vi "Run.vi"(9 "Team In":refnum<class "Team.lvclass">, 11 "MySquare in":refnum<class "MySquare.lvclass">) -> (1 "Team":refnum<class "Team.lvclass">, 2 "Run Result":T1={"Action"=enum."Move", "Direction"=enum."NW", "Replication"=refnum}, 3 "Square out":refnum<class "Square.lvclass">)   [LabVIEW 2020, in "The_Hill_Youth.lvlib" / "MySquare.lvclass"]
doc: "This VI is called on every active square each turn of the game for the square to decide what action to take."
uses:
  MySquare.lvclass
  C:/dev/lv20CE/sol-squarebattle/ProjectTemplates/Source/SummerOfLabVIEW/SquareBattle/template/SquareBattle/Square/Square.lvclass
  SquareBattle/Square/Square.lvclass
  SquareBattle/Run Result.ctl
  SquareBattle/Action.ctl
  SquareBattle/Direction.ctl
  SquareBattle/Team/Team.lvclass
  MyTeam/MyTeam.lvclass
  C:/dev/lv20CE/sol-squarebattle/ProjectTemplates/Source/SummerOfLabVIEW/SquareBattle/template/SquareBattle/Team/Team.lvclass
  SquareBattle/Square/Square.lvclass/Square.ctl
  MyTeam/map_point.ctl
  MySquare.lvclass/MySquare.ctl
  SquareBattle/Team/Team.lvclass/Team.ctl
  SquareBattle/SquareBattle.lvlib
  The_Hill_Youth.lvlib
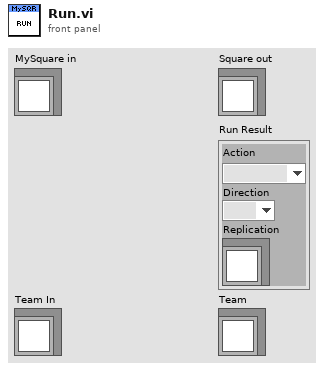
[diagram p1: front panel]
types:
  T1 = typedef "SquareBattle.lvlib/Run Result.ctl" = cluster{"Action":T2, "Direction":T3, "Replication":refnum<class "Square.lvclass">}
  T2 = typedef "SquareBattle.lvlib/Action.ctl" = enum16{"Wait", "Move", "Attack", "Replicate"}
  T3 = typedef "SquareBattle.lvlib/Direction.ctl" = enum16{"NW", "N", "NE", "E", "SE", "S", "SW", "W"}
  T4 = typedef "The_Hill_Youth.lvlib/map_point.ctl" = cluster{"status":enum16{"unknown", "frind", "enemy", "empty"}, "plans":enum16{"stay", "duplicate", "attack", "move to", "no plans"}, "age":dbl}
  T5 = typedef "SquareBattle.lvlib/Position.ctl" = cluster{"Row":i32, "Col":i32}
  T6 = enum16{"stay", "duplicate", "attack", "move to", "no plans"}
  T7 = typedef "SquareBattle.lvlib/Team Stats.ctl" = cluster{"Active":i32, "Generated":i32, "Kills":i32, "Eliminated":i32, "Collided":i32}
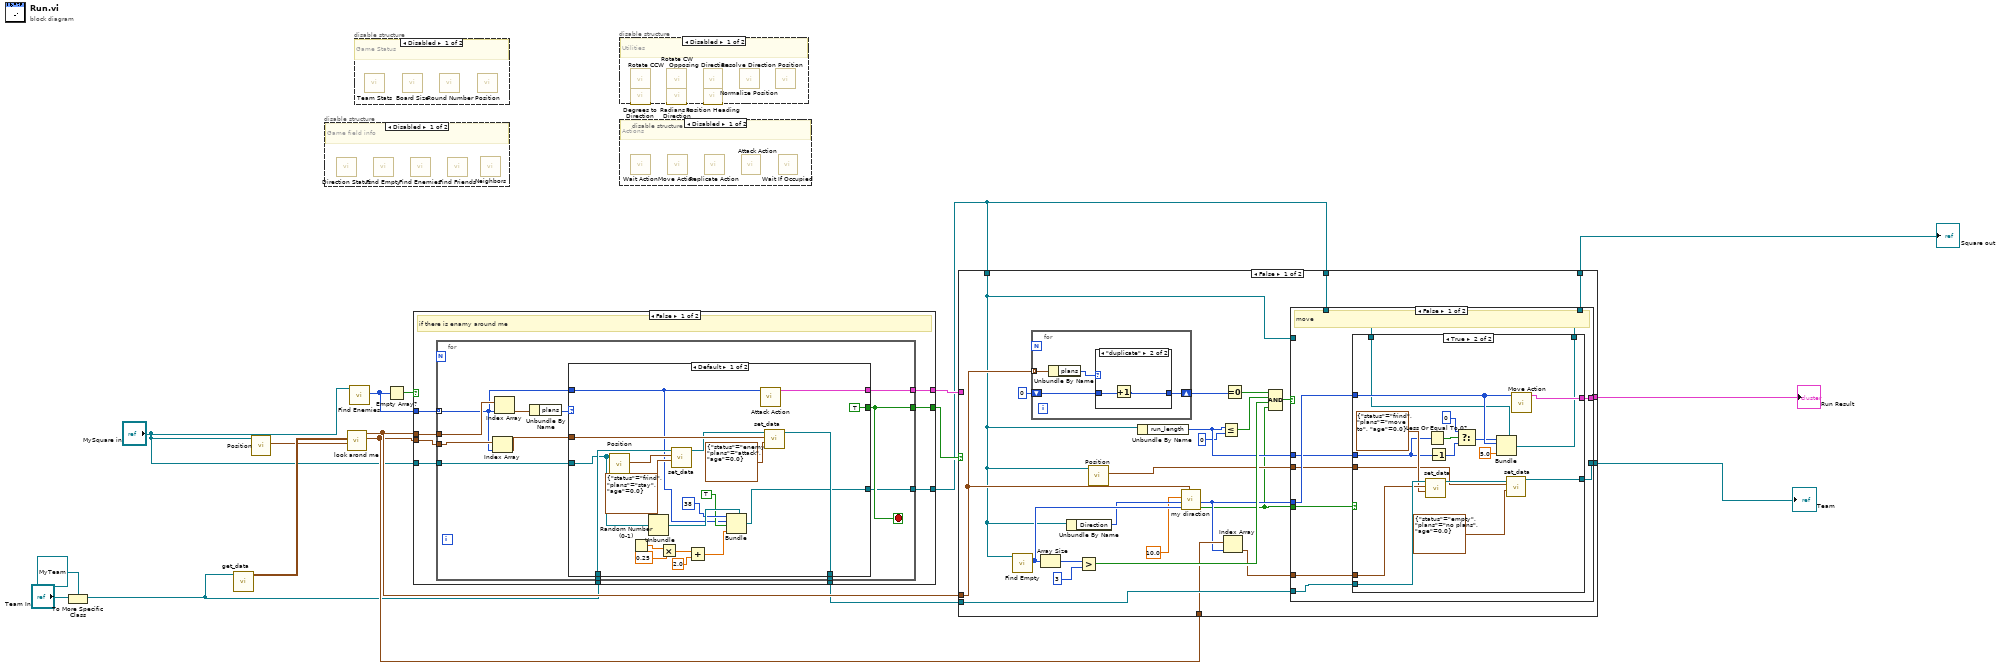
[diagram p0: block diagram]
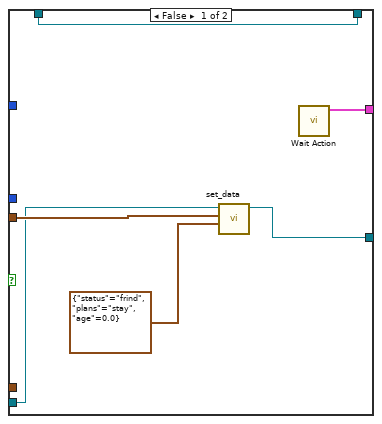
[diagram p2: hidden frame]
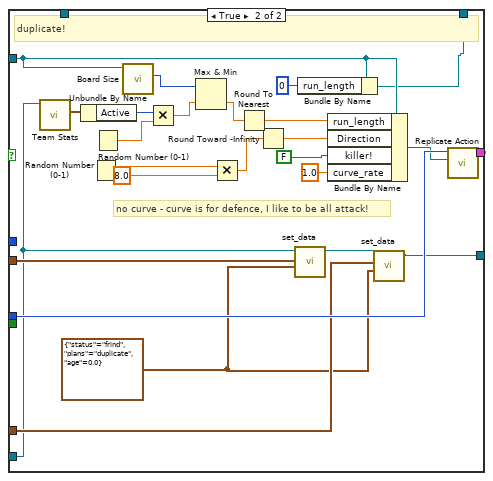
[diagram p3: hidden frame]
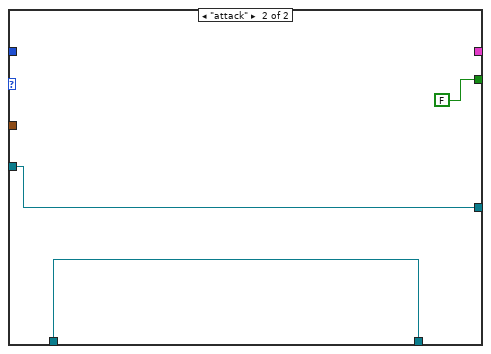
[diagram p6: hidden frame]
diagram:
  n1 = To More Specific Class(target class=refnum<class "MyTeam.lvclass"> refnum ("SquareTeam.lvlib:MyTeam.lvclass"), reference="Team In") -> (specific class reference=w7:refnum<class "MyTeam.lvclass">)  [unwired: 1 in, 1 out]
  n2 = call "get_data.vi"("SquareTeam.lvlib:MyTeam.lvclass"=w7) -> ("map"=w15:T4[][])  [unwired: 9 in, 1 out]
  n3 = call "Position.vi"("Square in"="MySquare in") -> ("Position"=w4:T5)  [unwired: 10 in]
  n4 = disable-structure shown="Disabled" {
    frame Disabled {
      # "Game field info"
      n5 = call "Direction Status.vi"() -> ()  [unwired: 10 in, 2 out]
      n6 = call "Find Empty.vi"() -> ()  [unwired: 11 in, 1 out]
      n7 = call "Find Enemies.vi"() -> ()  [unwired: 11 in, 1 out]
      n8 = call "Find Friends.vi"() -> ()  [unwired: 11 in, 1 out]
      n9 = call "Neighbors.vi"() -> ()  [unwired: 11 in, 1 out]
    }
    frame Enabled {
    }
  }
  n10 = call "look arond me.vi"("Position"=w4, "map"=w15) -> ("index_out"=w8:cluster{"Numeric":i32, "Numeric":i32}[], "map data of it"=w11:T4[])  [unwired: 8 in]
  n11 = call "Find Enemies.vi"("Square"="MySquare in") -> ("Enemy Directions"=w13:T3[])  [unwired: 10 in]
  n12 = disable-structure shown="Disabled" {
    frame Disabled {
      # "Game Status"
      n13 = call "Team Stats.vi"() -> ()  [unwired: 11 in, 1 out]
      n14 = call "Board Size.vi"() -> ()  [unwired: 11 in, 1 out]
      n15 = call "Round Number.vi"() -> ()  [unwired: 11 in, 1 out]
      n16 = call "Position.vi"() -> ()  [unwired: 11 in, 1 out]
    }
    frame Enabled {
    }
  }
  n17 = Empty Array?(array=w13) -> (empty?=w14:bool)
  n18 = case shown="False" w14 {
    tunnel: w13 -> [w26 _]
    tunnel: w11 -> [w25 _]
    tunnel: w8 -> [w24 _]
    tunnel: w7 -> [w23 w62]
    tunnel: [w22 _] -> w12
    tunnel: [w21 _] -> w10
    tunnel: [w20 w62] -> w9
    tunnel: "MySquare in" -> [w19 w61]
    tunnel: [w18 w61] -> w5
    frame False {
      # "if there is enamy around me"
      n19 = for {
        tunnel: w26 -> [w34] mode=indexing
        tunnel: w25 -> [w38]
        tunnel: w24 -> [w35]
        tunnel: w23 -> [w32]
        tunnel: [w31] -> w22
        tunnel: [w30] -> w21
        tunnel: [w29] -> w20
        tunnel: w19 -> [w27]
        tunnel: [w28] -> w18
        stop <- w30 stop-if-true
        n20 = Index Array(array=w35, index=w34) -> (element=w33:cluster{"Numeric":i32, "Numeric":i32})
        n21 = Index Array(array=w38, index=w34) -> (element=w37:T4)
        n22 = Unbundle By Name(w37) -> ("plans"=w36:T6)
        n23 = case shown="Default" w36 {
          tunnel: [TRUE FALSE] -> w30
          tunnel: w34 -> [w44 _]
          tunnel: [w56 _] -> w31
          tunnel: w33 -> [w55 _]
          tunnel: w32 -> [w53 w59]
          tunnel: [w49 w59] -> w29
          tunnel: w27 -> [w48 w58]
          tunnel: [w47 w58] -> w28
          frame Default {
            n24 = call "Position.vi"("Square in"=w48) -> ("Position"=w51:T5)  [unwired: 10 in]
            n25 = Random Number (0-1)() -> (number: 0 to 1=w43:dbl)
            n26 = Unbundle(w48) -> ()  [unwired: 4 out]
            n27 = Multiply(x=w43, y=0.25) -> (x*y=w42:dbl)
            n28 = call "set_data.vi"("new data"=T4 {"status"=enum."frind", "plans"=enum."stay", "age"=0.0}, "point to set index"=w51, "SquareTeam.lvlib:MyTeam.lvclass 2"=w53) -> ("SquareTeam.lvlib:MyTeam.lvclass"=w52:refnum<class "MyTeam.lvclass">)  [unwired: 8 in]
            n29 = Add(x=w42, y=2.0) -> (x+y=w40:dbl)
            n30 = Bundle(cluster=w48, 38 ("x"), w44, TRUE ("killer!"), w40) -> (w47:refnum<class "MySquare.lvclass">)
            n31 = call "Attack Action.vi"("Direction"=w44) -> ("Run Result"=w56:T1)  [unwired: 10 in]
            n32 = call "set_data.vi"("new data"=T4 {"status"=enum."enemy", "plans"=enum."attack", "age"=0.0}, "point to set index"=w55, "SquareTeam.lvlib:MyTeam.lvclass 2"=w52) -> ("SquareTeam.lvlib:MyTeam.lvclass"=w49:refnum<class "MyTeam.lvclass">)  [unwired: 8 in]
          }
          frame "attack" {
          }
        }
      }
    }
    frame True {
    }
  }
  n33 = disable-structure shown="Disabled" {
    frame Disabled {
      # "Utilities"
      n34 = call "Rotate CCW.vi"() -> ()  [unwired: 11 in, 1 out]
      n35 = call "Degrees to Direction.vi"() -> ()  [unwired: 11 in, 1 out]
      n36 = call "Rotate CW.vi"() -> ()  [unwired: 11 in, 1 out]
      n37 = call "Radians to Direction.vi"() -> ()  [unwired: 11 in, 1 out]
      n38 = call "Opposing Direction.vi"() -> ()  [unwired: 11 in, 1 out]
      n39 = call "Position Heading.vi"() -> ()  [unwired: 10 in, 2 out]
      n40 = call "Normalize Position.vi"() -> ()  [unwired: 10 in, 2 out]
      n41 = call "Resolve Direction Position.vi"() -> ()  [unwired: 9 in, 3 out]
    }
    frame Enabled {
    }
  }
  n42 = disable-structure shown="Disabled" {
    frame Disabled {
      # "Actions"
      n43 = call "Wait Action.vi"() -> ()  [unwired: 11 in, 1 out]
      n44 = call "Move Action.vi"() -> ()  [unwired: 11 in, 1 out]
      n45 = call "Replicate Action.vi"() -> ()  [unwired: 11 in, 1 out]
      n46 = call "Attack Action.vi"() -> ()  [unwired: 11 in, 1 out]
      n47 = call "Wait If Occupied.vi"() -> ()  [unwired: 11 in, 1 out]
    }
    frame Enabled {
    }
  }
  n48 = case shown="False" w10 {
    tunnel: w12 -> [_ w155]
    tunnel: [w77 w155] -> w3
    tunnel: w11 -> [w84 _]
    tunnel: w5 -> [w65 _]
    tunnel: w9 -> [w76 w154]
    tunnel: w5 -> [w75 w153]
    tunnel: w8 -> [w73 _]
    tunnel: [w71 w154] -> w6
    tunnel: [w70 w153] -> w1
    frame False {
      n49 = call "Find Empty.vi"("Square"=w65) -> ("Empty Directions"=w85:T3[])  [unwired: 10 in]
      n50 = for {
        tunnel: w84 -> [w149] mode=indexing
        shift-right: [w147] -> w82
        shift-left: u8 0 -> [w146]
        n51 = Unbundle By Name(w149) -> ("plans"=w148:T6)
        n52 = case shown="\"duplicate\"" w148 {
          tunnel: [w150 w152] -> w147
          tunnel: w146 -> [w150 w151]
          frame "stay", Default {
          }
          frame "duplicate" {
            n53 = Increment(x=w151) -> (x+1=w152:u8)
          }
        }
      }
      n54 = Array Size(array=w85) -> (size(s)=w87:i32)
      n55 = Unbundle By Name(w65) -> ("Direction"=w66:T3)
      n56 = Greater?(x=w87, y=3) -> (0:w79:bool)
      n57 = call "Position.vi"("Square in"=w65) -> ("Position"=w74:T5)  [unwired: 10 in]
      n58 = Unbundle By Name(w65) -> ("run_length"=w69:i32)
      n59 = call "my diraction.vi"(7:w84, "Empty Directions"=w85, "my diraction"=w66, "curve_rate"=10.0) -> ("you may act"=w64:bool, "Direction for act"=w67:i16)  [unwired: 5 in, 1 out]
      n60 = Less Or Equal?(x=w69, y=0) -> (x <= y?=w80:bool)
      n61 = Index Array(array=w73, index=w67) -> (element=w72:cluster{"Numeric":i32, "Numeric":i32})
      n62 = Equal To 0?(x=w82) -> (x = 0?=w81:bool)
      n63 = Compound Arithmetic op=AND(w81, w80, w79, w64) -> (w78:bool)
      n64 = case shown="False" w78 {
        tunnel: w67 -> [w96 w145]
        tunnel: [w95 w144] -> w77
        tunnel: w76 -> [w94 w130]
        tunnel: w75 -> [w89 _]
        tunnel: w74 -> [w91 w141]
        tunnel: w72 -> [w93 w139]
        tunnel: [w92 w137] -> w71
        tunnel: w64 -> [w97 _]
        tunnel: w69 -> [w90 _]
        tunnel: [w88 w124] -> w70
        tunnel: w65 -> [_ w125]
        frame False {
          # "move"
          n65 = case shown="True" w97 {
            tunnel: w96 -> [_ w111]
            tunnel: [w99 w120] -> w95
            tunnel: w94 -> [w102 w119]
            tunnel: w93 -> [_ w118]
            tunnel: [w100 w115] -> w92
            tunnel: w91 -> [w103 w114]
            tunnel: w90 -> [_ w110]
            tunnel: w89 -> [w98 w105]
            tunnel: [w98 w112] -> w88
            frame False {
              n66 = call "set_data.vi"("new data"=T4 {"status"=enum."frind", "plans"=enum."stay", "age"=0.0}, "point to set index"=w103, "SquareTeam.lvlib:MyTeam.lvclass 2"=w102) -> ("SquareTeam.lvlib:MyTeam.lvclass"=w100:refnum<class "MyTeam.lvclass">)  [unwired: 8 in]
              n67 = call "Wait Action.vi"() -> ("Run Result"=w99:T1)  [unwired: 11 in]
            }
            frame True {
              # "move!"
              n68 = call "set_data.vi"("new data"=T4 {"status"=enum."frind", "plans"=enum."move to", "age"=0.0}, "point to set index"=w118, "SquareTeam.lvlib:MyTeam.lvclass 2"=w119) -> ("SquareTeam.lvlib:MyTeam.lvclass"=w116:refnum<class "MyTeam.lvclass">)  [unwired: 8 in]
              n69 = Less Or Equal To 0?(x=w110) -> (x <= 0?=w108:bool)
              n70 = Decrement(x=w110) -> (x-1=w109:i32)
              n71 = Select(t=0, s=w108, f=w109) -> (s? t:f=w106:i32)
              n72 = Bundle(cluster=w105, w106, w111, 5.0 ("curve_rate")) -> (w112:refnum<class "MySquare.lvclass">)  [unwired: 1 in]
              n73 = call "set_data.vi"("new data"=T4 {"status"=enum."empty", "plans"=enum."no plans", "age"=0.0}, "point to set index"=w114, "SquareTeam.lvlib:MyTeam.lvclass 2"=w116) -> ("SquareTeam.lvlib:MyTeam.lvclass"=w115:refnum<class "MyTeam.lvclass">)  [unwired: 8 in]
              n74 = call "Move Action.vi"("Direction"=w111) -> ("Run Result"=w120:T1)  [unwired: 10 in]
            }
          }
        }
        frame True {
          w138 = T4 {"status"=enum."frind", "plans"=enum."duplicate", "age"=0.0} ("new data")
          # "no curve - curve is for defence, I like to be all attack!"
          # "duplicate!"
          n75 = call "Team Stats.vi"("Team"=w130) -> ("Team Stats"=w143:T7)  [unwired: 10 in]
          n76 = Unbundle By Name(w143) -> ("Active"=w123:i32)
          n77 = Random Number (0-1)() -> (number: 0 to 1=w136:dbl)
          n78 = Random Number (0-1)() -> (number: 0 to 1=w142:dbl)
          n79 = call "Board Size.vi"("Square in"=w125) -> ("Board Size"=w132:i32)  [unwired: 10 in]
          n80 = Multiply(x=w123, y=w142) -> (x*y=w122:dbl)
          n81 = Max & Min(x=w132, y=w122) -> (min(x,y)=w121:dbl)  [unwired: 1 out]
          n82 = Multiply(x=w136, y=8.0) -> (x*y=w134:dbl)
          n83 = Round To Nearest(number=w121) -> (nearest integer value=w129:dbl)
          n84 = Round Toward -Infinity(1:w134) -> (0:w133:dbl)
          n85 = call "set_data.vi"("new data"=w138, "point to set index"=w141, "SquareTeam.lvlib:MyTeam.lvclass 2"=w130) -> ("SquareTeam.lvlib:MyTeam.lvclass"=w140:refnum<class "MyTeam.lvclass">)  [unwired: 8 in]
          n86 = Bundle By Name(cluster=w125, "run_length"=0) -> (w124:refnum<class "MySquare.lvclass">)
          n87 = Bundle By Name(cluster=w125, "run_length"=w129, "Direction"=w133, "killer!"=FALSE, "curve_rate"=1.0) -> (w127:refnum<class "MySquare.lvclass">)
          n88 = call "set_data.vi"("new data"=w138, "point to set index"=w139, "SquareTeam.lvlib:MyTeam.lvclass 2"=w140) -> ("SquareTeam.lvlib:MyTeam.lvclass"=w137:refnum<class "MyTeam.lvclass">)  [unwired: 8 in]
          n89 = call "Replicate Action.vi"("Square Type"=w127, "Direction"=w145) -> ("Run Result"=w144:T1)  [unwired: 9 in]
        }
      }
    }
    frame True {
      # "if he alrady attack - just do it"
    }
  }
  "Square out" <- w1
  "Run Result" <- w3
  "Team" <- w6
